vi "Set image colour.vi"(8 "error in":errorcluster) -> (0 "error out":errorcluster)   [LabVIEW 2017]
uses:
  Timelapse Viewer/Globals/gl_Time series viewer globals.vi
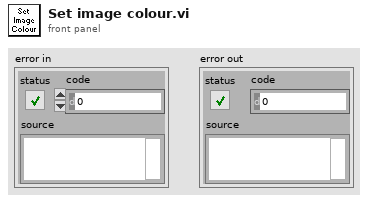
[diagram p1: front panel]
types:
  T1 = typedef "Time series viewer refs.ctl" = cluster{"This VI":refnum<vi>, "Image control":refnum<vi>, "AVI Mode ind":refnum<vi>, "Play":refnum<vi>, "Stop":refnum<vi>, "Back":refnum<vi>, "Scrollbar":refnum<vi>, "Video length info":refnum<vi>, "Expected speed values":refnum<vi>, "Intensity":refnum<vi>, "Path":refnum<vi>, "Selection sliders":refnum<vi>, "Speed Graph ref":refnum<vi>, "Frame rate set (fps)":refnum<vi>, "Channel to load":refnum<vi>, "Number of rows to generate":refnum<vi>, "Colour":refnum<vi>}
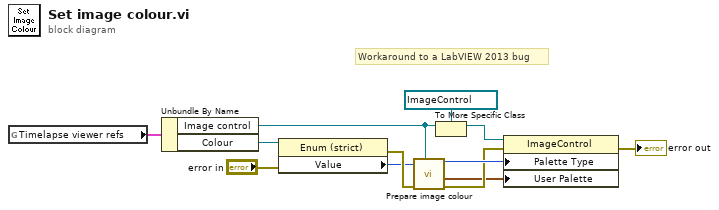
[diagram p0: block diagram]
diagram:
  # "Workaround to a LabVIEW 2013 bug"
  n1 = global read "gl_Time series viewer globals.vi" "Timelapse viewer refs"() -> (w2:T1)
  n2 = Unbundle By Name(w2) -> ("Image control"=w9:refnum<vi>, "Colour"=w3:refnum<vi>)
  n3 = property class="Enum (strict)"(reference=w3, error in="error in") -> (error out=w5:errorcluster, "Value"=w1:enum16{"Gray", "Red", "Green"})  [unwired: 1 out]
  n4 = call "Prepare image colour.vi"("Image control"=w9, "error in"=w5, "Left Image Palette"=w1) -> ("error out"=w6:errorcluster, "Color Palette"=w4:cluster{"Red":u8, "Green":u8, "Blue":u8}[], "Palette Type"=w7:u32)  [unwired: 6 in]
  n5 = To More Specific Class(target class=refnum<vi> refnum ("Image"), reference=w9) -> (specific class reference=w10:refnum<vi>)  [unwired: 1 in, 1 out]
  n6 = property on="Property Node" class="ImageControl"(reference=w10, error in=w6, "Palette Type"=w7, "User Palette"=w4) -> (error out=→"error out":errorcluster)  [unwired: 1 out]
